vi "Pass-Fail.vi"(6 "Counts in":T1, 8 "error in":errorcluster, 9 "Completed? in":bool, 10 "Results in":T3, 11 "Results Cluster in":T2) -> (0 "error out":errorcluster, 1 "Completed? out":bool, 2 "Results out":T3, 4 "Counts out":T1)   [LabVIEW 2017]
uses:
  controls/AC Results.ctl
  controls/Results Cluster.ctl
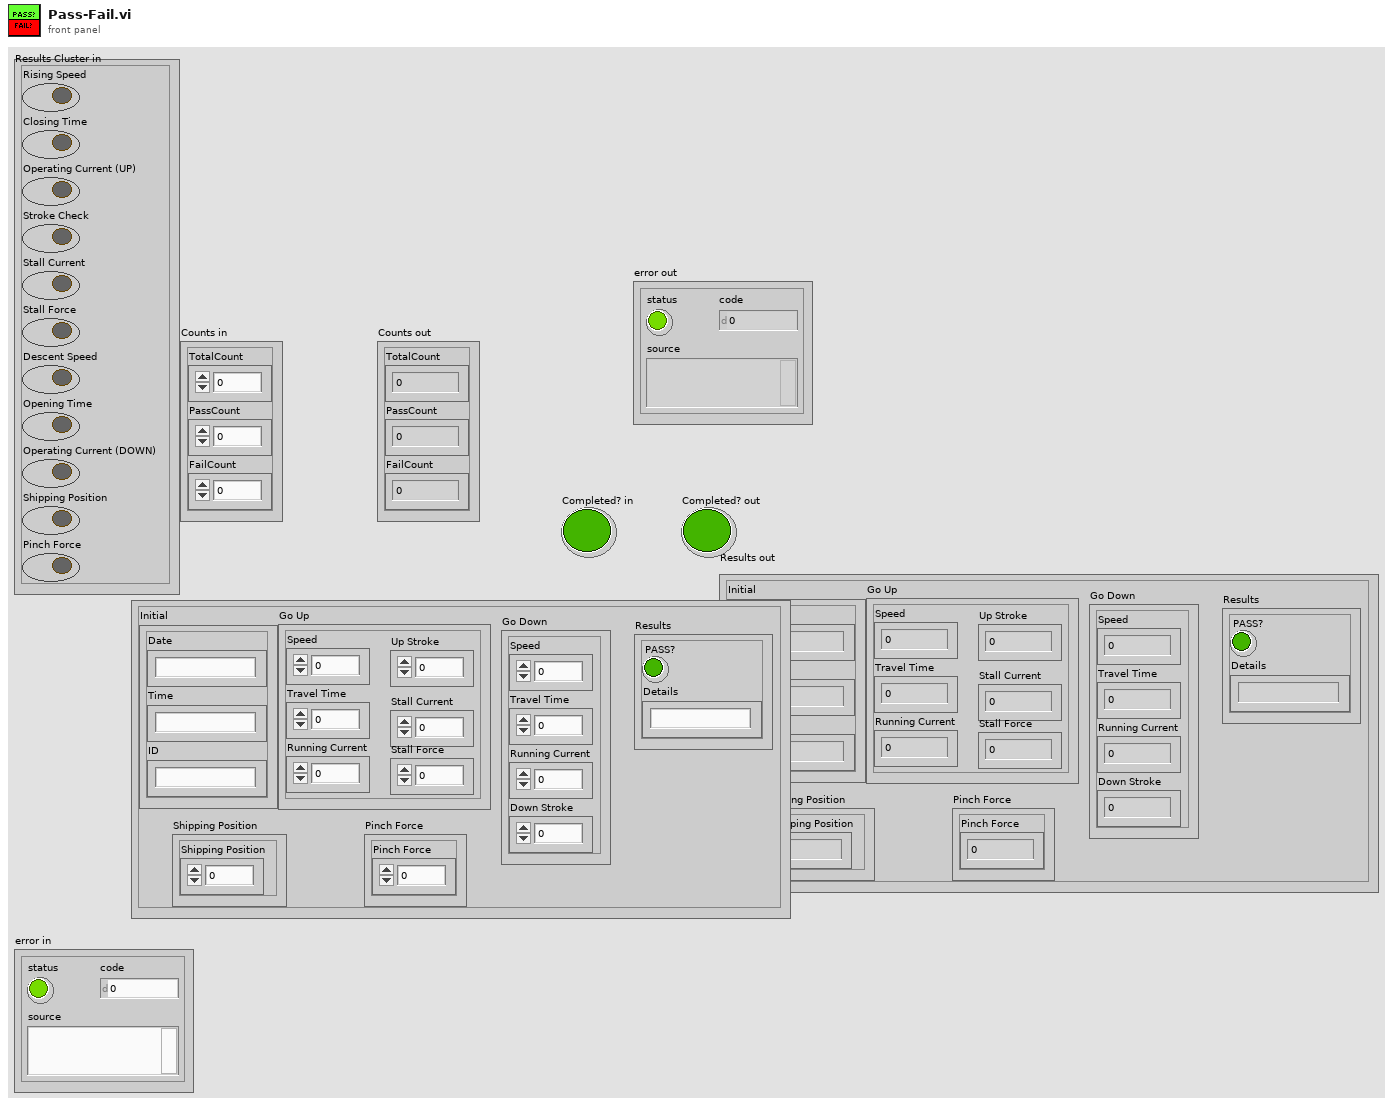
[diagram p1: front panel]
types:
  T1 = cluster{"TotalCount":u16, "PassCount":u16, "FailCount":u16}
  T2 = typedef "Results Cluster.ctl" = cluster{"Rising Speed":bool, "Closing Time":bool, "Operating Current (UP)":bool, "Stroke Check":bool, "Stall Current":bool, "Stall Force":bool, "Descent Speed":bool, "Opening Time":bool, "Operating Current (DOWN)":bool, "Shipping Position":bool, "Pinch Force":bool}
  T3 = typedef "AC Results.ctl" = cluster{"Initial":cluster{"Date":string, "Time":string, "ID":string}, "Go Up":cluster{"Speed":dbl, "Travel Time":dbl, "Running Current":dbl, "Up Stroke":dbl, "Stall Current":dbl, "Stall Force":dbl}, "Go Down":cluster{"Speed":dbl, "Travel Time":dbl, "Running Current":dbl, "Down Stroke":dbl}, "Shipping Position":cluster{"Shipping Position":dbl}, "Results":cluster{"PASS?":bool, "Details":string}, "Pinch Force":cluster{"Pinch Force":dbl}}
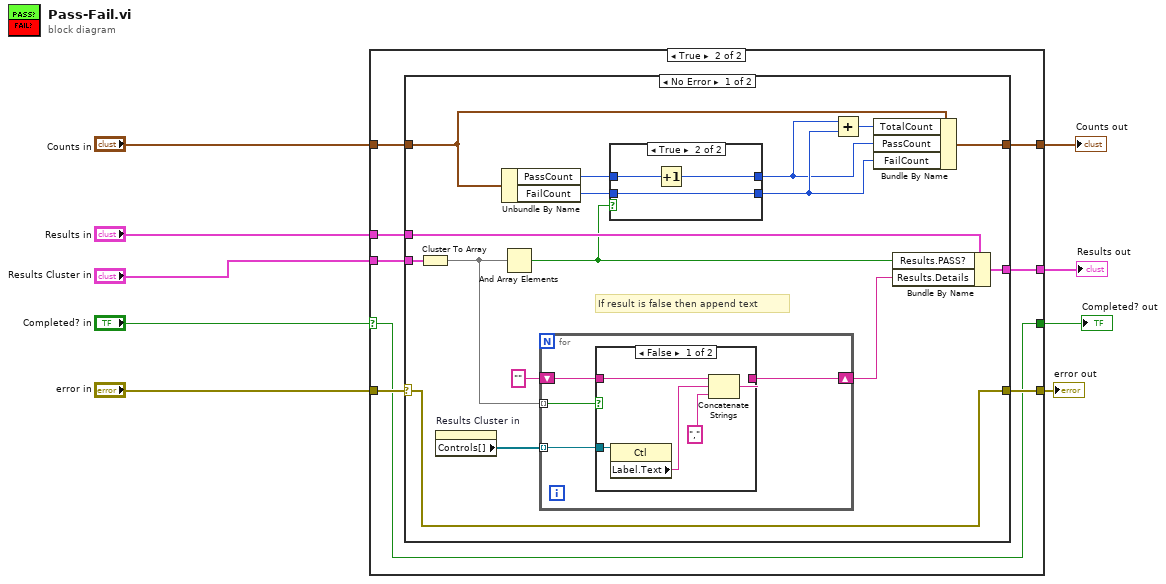
[diagram p0: block diagram]
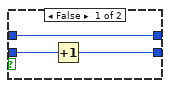
[diagram p3: hidden frame]
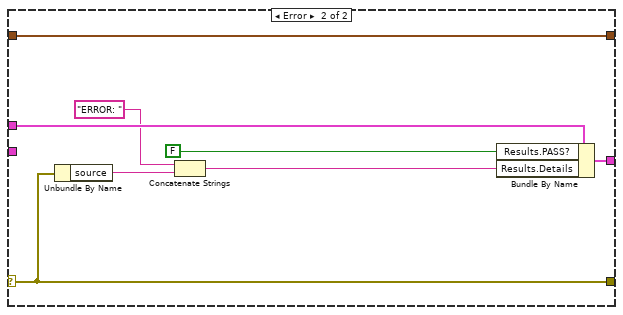
[diagram p5: hidden frame]
diagram:
  n1 = case shown="True" "Completed? in" {
    selector: "Completed? in" -> [w10 w14]
    tunnel: "error in" -> [w11 w21]
    tunnel: "Results in" -> [w12 w20]
    tunnel: "Results Cluster in" -> [_ w19]
    tunnel: "Counts in" -> [w13 w18]
    tunnel: [w13 w17] -> w5
    tunnel: [w12 w16] -> w4
    tunnel: [w11 w15] -> w2
    tunnel: [w10 w14] -> w1
    frame False {
    }
    frame True {
      n2 = case shown="No Error" w21 {
        selector: w21 -> [w22 w57]
        tunnel: w19 -> [w37 _]
        tunnel: w20 -> [w36 w61]
        tunnel: [w35 w60] -> w16
        tunnel: w18 -> [w30 w58]
        tunnel: [w25 w58] -> w17
        tunnel: [w22 w57] -> w15
        frame No Error {
          # "If result is false then append text"
          n3 = Cluster To Array(cluster=w37) -> (array=w32:bool[])
          n4 = property on="Results Cluster in" class="Clust (strict)"() -> ("Controls[]"=w34:refnum<vi>[])  [unwired: 2 in, 2 out]
          n5 = Unbundle By Name(w30) -> ("PassCount"=w26:u16, "FailCount"=w27:u16)
          n6 = And Array Elements(Boolean array=w32) -> (logical AND=w28:bool)
          n7 = for {
            tunnel: w32 -> [w46] mode=indexing
            tunnel: w34 -> [w47] mode=indexing
            shift-right: [w44] -> w31
            shift-left: "" -> [w45]
            n8 = case shown="False" w46 {
              tunnel: w47 -> [w52 _]
              tunnel: w45 -> [w50 w53]
              tunnel: [w49 w53] -> w44
              frame False {
                n9 = property class="Ctl"(reference=w52) -> ("Label.Text"=w51:string)  [unwired: 1 in, 2 out]
                n10 = Concatenate Strings(w50, w51, ",") -> (w49:string)
              }
              frame True {
              }
            }
          }
          n11 = case shown="True" w28 {
            tunnel: w27 -> [w39 w43]
            tunnel: [w38 w43] -> w24
            tunnel: w26 -> [w40 w42]
            tunnel: [w40 w41] -> w23
            frame False {
              n12 = Increment(x=w39) -> (x+1=w38:u16)
            }
            frame True {
              n13 = Increment(x=w42) -> (x+1=w41:u16)
            }
          }
          n14 = Add(x=w23, y=w24) -> (x+y=w29:u16)
          n15 = Bundle By Name(cluster=w30, "TotalCount"=w29, "PassCount"=w23, "FailCount"=w24) -> (w25:T1)
          n16 = Bundle By Name(cluster=w36, "Results.PASS?"=w28, "Results.Details"=w31) -> (w35:T3)
        }
        frame Error {
          n17 = Unbundle By Name(w57) -> ("source"=w55:string)
          n18 = Concatenate Strings("ERROR: " ("string"), w55) -> (w54:string)
          n19 = Bundle By Name(cluster=w61, "Results.PASS?"=FALSE, "Results.Details"=w54) -> (w60:T3)
        }
      }
    }
  }
  "Counts out" <- w5
  "Results out" <- w4
  "error out" <- w2
  "Completed? out" <- w1
